vi "Optris_demo.vi"() -> ()   [LabVIEW 2019]
uses:
  <vilib>/Instr/_visa.llb/VISA Configure Serial Port (Instr).vi
panel:
  out "?":waveform(dbl)(graph)
  out "Calibration":u32
  out "Data->Decimal":u32
  out "Buffer":string
  in  "정지":bool
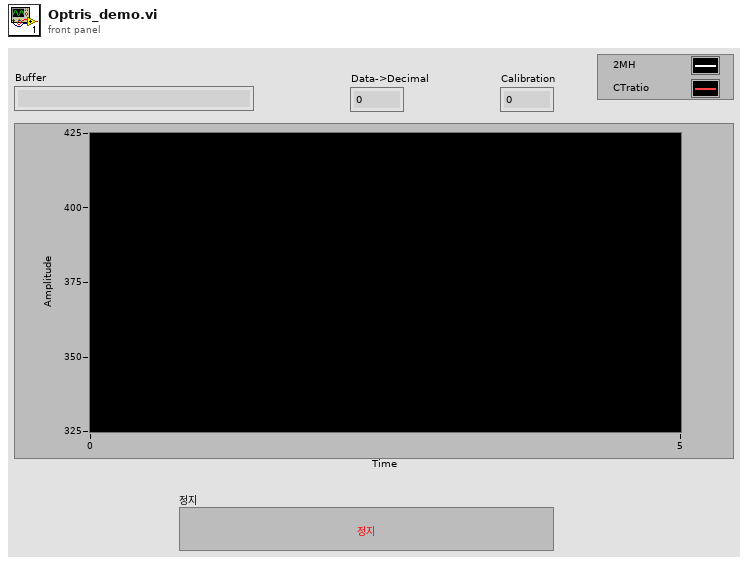
[diagram p1: front panel]
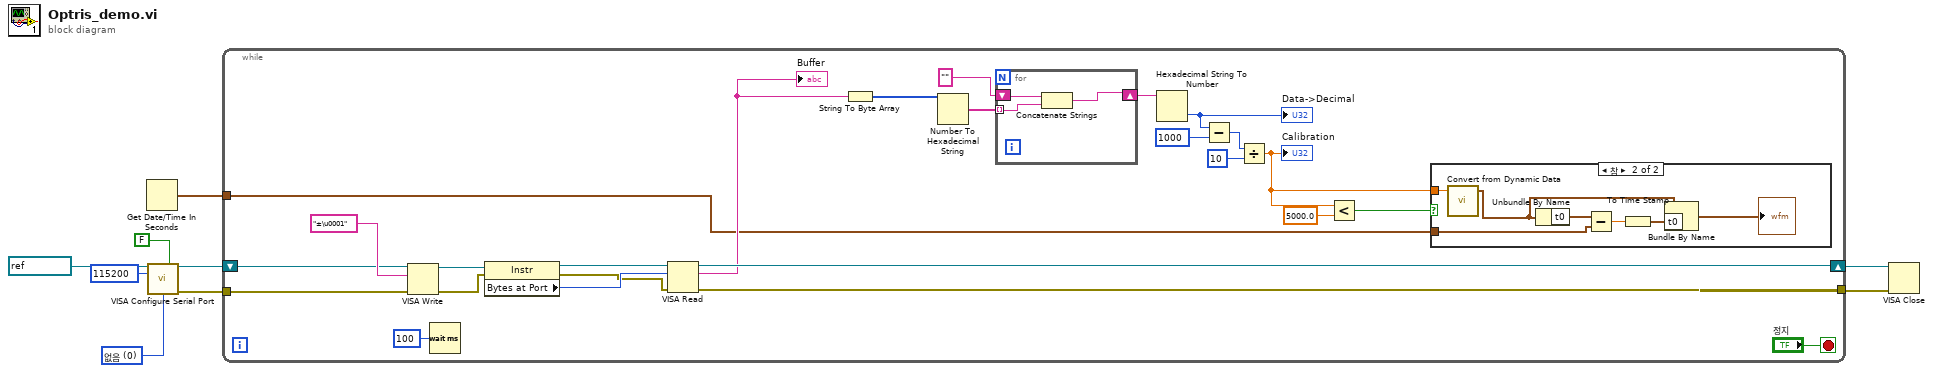
[diagram p0: block diagram]
diagram:
  w5 = u16 0 items=["없음", "XON/XOFF", "RTS/CTS", "XON/XOFF & RTS/CTS", "DTR/DSR", "XON/XOFF & DTR/DSR"] ("flow control (0:none)")
  n1 = Get Date/Time In Seconds() -> (seconds since 1Jan1904=w1:timestamp)
  n2 = call-poly "VISA Configure Serial Port"("VISA resource name"=refnum<visa-resource-name> "COM7", "Enable Termination\nChar (T)"=FALSE ("Enable Termination\nChar (T)"), "baud rate (9600)"=u32 115200, "flow control (0:none)"=w5) -> ("VISA resource name out"=w4:refnum<visa-resource-name>, "error out"=w3:errorcluster)  [unwired: 10 in]
  n3 = while {
    shift-right: [w28] -> w7
    shift-left: w4 -> [w17]
    tunnel: w3 -> [w34]
    tunnel: [w14] -> w2
    tunnel: w1 -> [w13]
    stop <- "정지" stop-if-true
    n4 = VISA Write(VISA resource name=w17, write buffer="±\u0001" ("버퍼 쓰기"), error in (no error)=w34) -> (VISA resource name out=w33:refnum<visa-resource-name>, error out=w32:errorcluster)  [unwired: 1 out]
    n5 = Wait (ms)(milliseconds to wait=u32 100 ("대기 시간 (ms)")) -> ()  [unwired: 1 out]
    n6 = property class="Instr"(reference=w33, error in=w32) -> (reference out=w30:refnum<visa-resource-name>, error out=w16:errorcluster, "Bytes at Port"=w29:u32)
    n7 = VISA Read(VISA resource name=w30, byte count=w29, error in (no error)=w16) -> (VISA resource name out=w28:refnum<visa-resource-name>, read buffer=w23:string, error out=w14:errorcluster)  [unwired: 1 out]
    "Buffer" <- w23
    n8 = String To Byte Array(string=w23) -> (unsigned byte array=w26:u8[])
    n9 = Number To Hexadecimal String(2:w26) -> (0:w25:string[])  [unwired: 1 in]
    n10 = for {
      tunnel: w25 -> [w43] mode=indexing
      shift-right: [w42] -> w15
      shift-left: "" -> [w44]
      n11 = Concatenate Strings(w44, w43) -> (w42:string)
    }
    n12 = Hexadecimal String To Number(string=w15) -> (number=w21:u32)  [unwired: 2 in, 1 out]
    "Data->Decimal" <- w21
    n13 = Subtract(x=w21, y=u32 1000) -> (x-y=w20:u32)
    n14 = Divide(x=w20, y=u32 10) -> (x/y=w11:dbl)
    "Calibration" <- w11
    n15 = Less?(x=w11, y=5000.0) -> (x < y?=w12:bool)
    n16 = case shown="참" w12 {
      tunnel: w11 -> [_ w41]
      tunnel: w13 -> [_ w35]
      frame False {
      }
      frame True {
        n17 = call "Convert from Dynamic Data"("Dynamic Data Type"=w41) -> ("Waveform"=w37:waveform(dbl))  [unwired: 3 in]
        n18 = Unbundle By Name(w37) -> ("t0"=w38:timestamp)
        n19 = Subtract(x=w38, y=w35) -> (x-y=w39:dbl)
        n20 = To Time Stamp(1:w39) -> (0:w40:timestamp)
        n21 = Bundle By Name(cluster=w37, "t0"=w40) -> (→"?":waveform(dbl))
      }
    }
  }
  n22 = VISA Close(VISA resource name=w7, error in (no error)=w2) -> ()  [unwired: 1 out]
